vi "Modules Selector.vi"(6 "Scan All":bool, 10 "DQMH Modules":T1[](array[typedef]), 11 "Project In":refnum<class "Project.lvclass">) -> (3 "Project Out":refnum<class "Project.lvclass">, 4 "Scan?":bool)   [LabVIEW 2019, in "Panther Dashboard.lvlib" / "Project.lvclass"]
uses:
  Project.lvclass
  Panther Dashboard/Module to scan--cluster.ctl
  <vilib>/Delacor/Delacor QMH/Libraries/Scripting API/Module Information--cluster.ctl
  Panther Dashboard/Module type--enum.ctl
  Library/Library.lvclass
  Library/Library.lvclass/Library.ctl
  Project.lvclass/Project.ctl
  Library/Write Library Ref.vi
  Library/Write Type.vi
  Library/Write Library Description.vi
  Library/Write Dependency.vi
  Write Libraries.vi
  Panther Dashboard/Panther Dashboard.lvlib
  <vilib>/Delacor/Delacor QMH/Libraries/Scripting API/DQMH_Scripting API.lvlib
panel:
  in  "DQMH Modules found in Project":T2[](array[typedef])
  in  "Scan Selection":bool
  in  "Select/Unselect All":bool
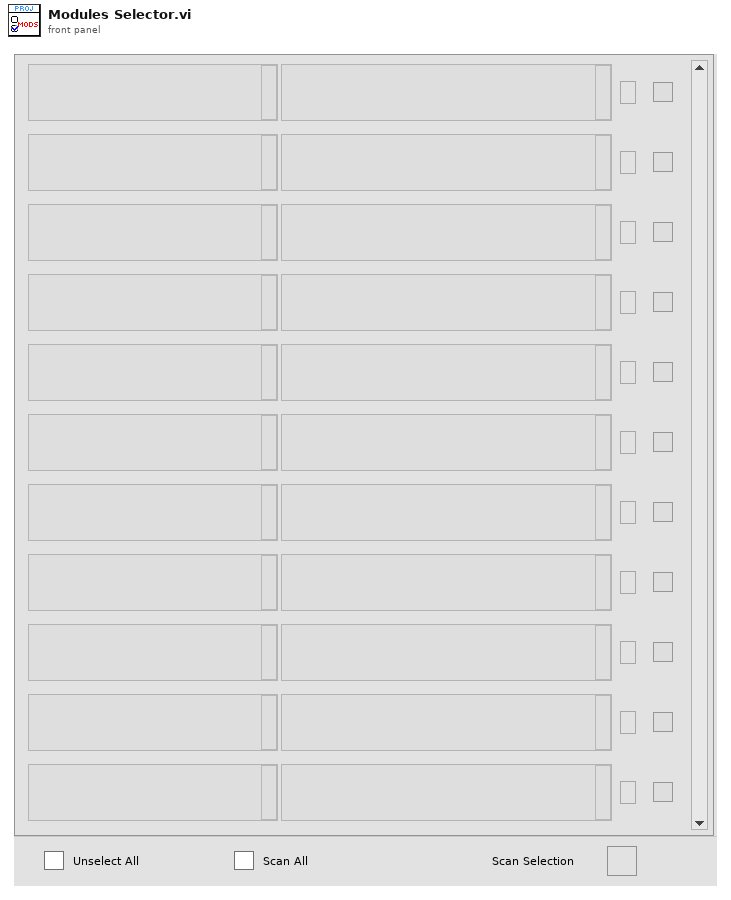
[diagram p1: front panel]
types:
  T1 = typedef "DQMH_Scripting API.lvlib/Module Information--cluster.ctl" = cluster{"Library":refnum<vi>, "Qualified Name":string, "Path":path, "Cloneable":bool, "Under Dependencies":bool}
  T2 = typedef "Panther Dashboard.lvlib/Module to scan--cluster.ctl" = cluster{"Module Name":string, "Description":string, "Scan?":bool, "Dependency":bool}
  T3 = typedef "Panther Dashboard.lvlib/Module type--enum.ctl" = enum16{"Singleton", "Cloneable"}
  T4 = enum32{"Invalid", "Standard", "Closed", "Hidden", "Minimized", "Maximized"}
  T5 = enum8{"Enabled", "Disabled", "Disabled and Grayed Out"}
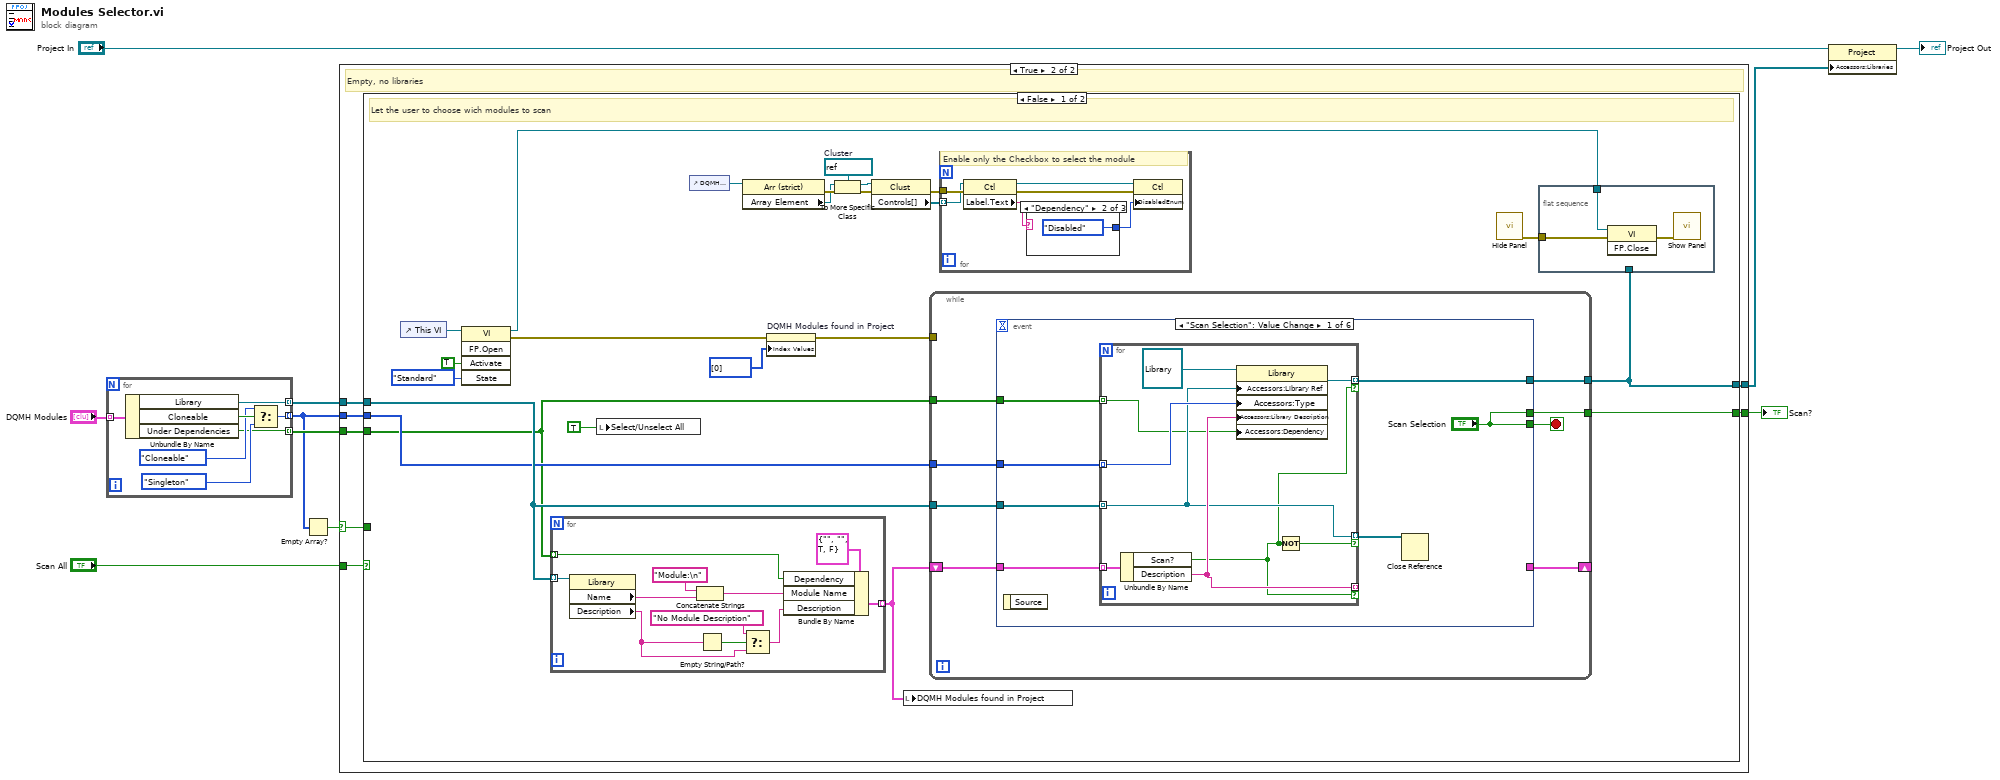
[diagram p0: block diagram]
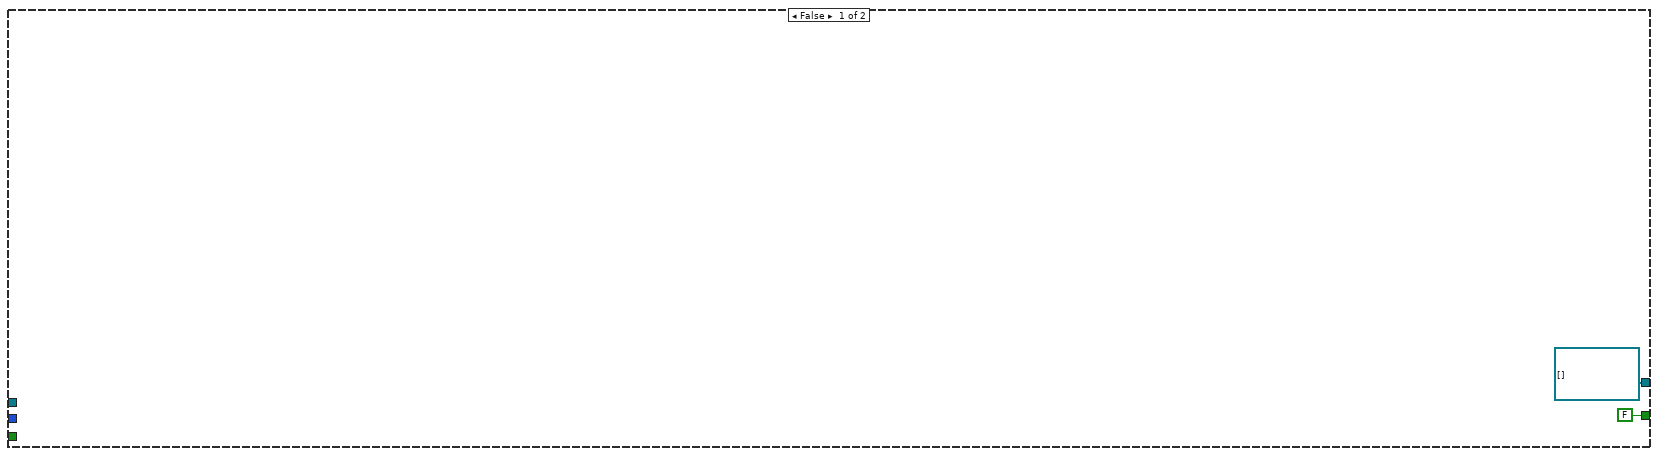
[diagram p2: hidden frame]
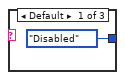
[diagram p3: hidden frame]
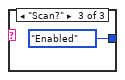
[diagram p4: hidden frame]
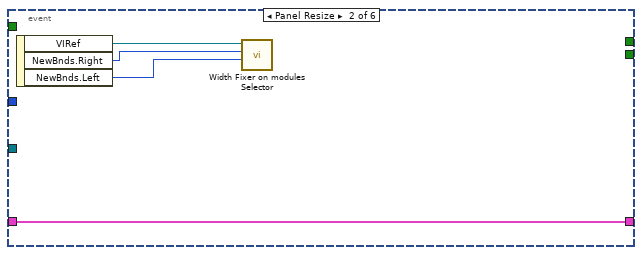
[diagram p5: hidden frame]
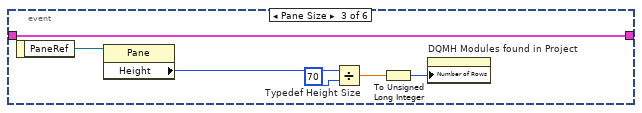
[diagram p6: hidden frame]
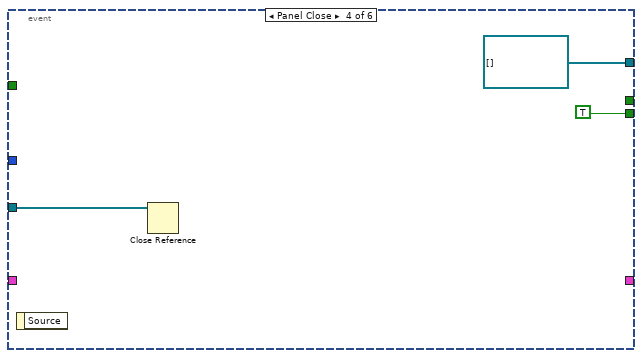
[diagram p7: hidden frame]
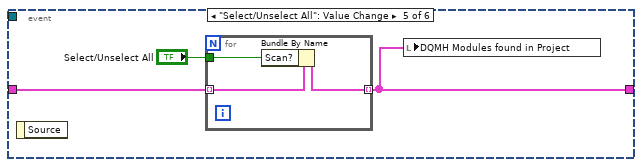
[diagram p8: hidden frame]
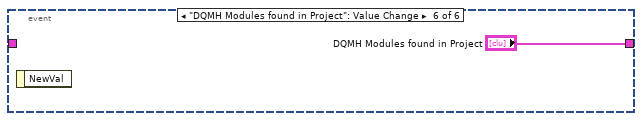
[diagram p9: hidden frame]
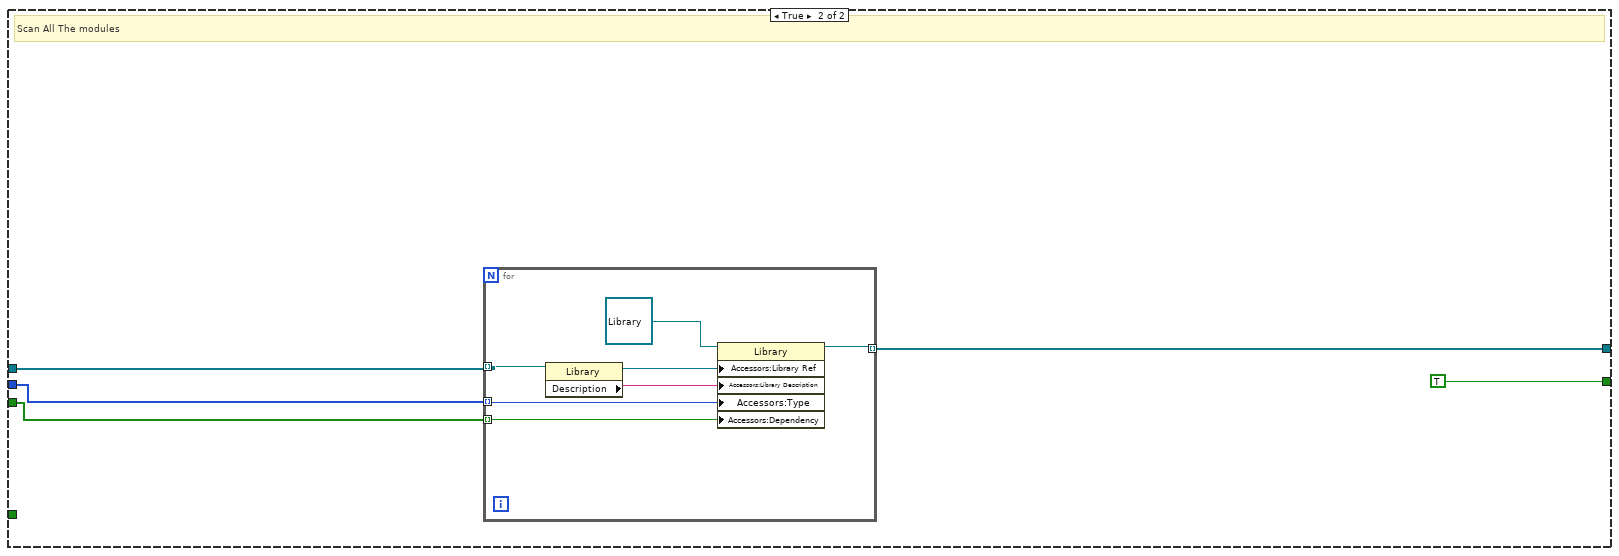
[diagram p10: hidden frame]
diagram:
  n1 = for {
    tunnel: "DQMH Modules" -> [w17] mode=indexing
    tunnel: [w16] -> w7 mode=indexing
    tunnel: [w12] -> w3 mode=indexing
    tunnel: [w11] -> w6 mode=indexing
    n2 = Unbundle By Name(w17) -> ("Library"=w16:refnum<vi>, "Cloneable"=w14:bool, "Under Dependencies"=w11:bool)
    n3 = Select(t=Module_type--enum."Cloneable", s=w14, f=Module_type--enum."Singleton" ("Module type")) -> (s? t:f=w12:T3)
  }
  n4 = Empty Array?(array=w3) -> (empty?=w4:bool)
  n5 = case shown="True" w4 {
    selector: w4 -> [_ w20]
    tunnel: [FALSE ("Scan Selection") w26] -> w10
    tunnel: "Scan All" -> [_ w25]
    tunnel: [refnum<class "Library.lvclass">[] [] w24] -> w8
    tunnel: w7 -> [_ w23]
    tunnel: w3 -> [_ w22]
    tunnel: w6 -> [_ w21]
    frame False {
    }
    frame True {
      # "Empty, no libraries"
      n6 = case shown="False" w25 {
        tunnel: w23 -> [w43 w120]
        tunnel: w22 -> [w42 w119]
        tunnel: w21 -> [w41 w118]
        tunnel: [w40 TRUE ("Scan Selection")] -> w26
        tunnel: [w27 w117] -> w24
        tunnel: w20 -> [_ _]
        frame False {
          w28 = refnum<vi> refnum  # Cluster
          # "Let the user to choose wich modules to scan"
          n7 = control-ref of="This VI"() -> (w39:refnum<vi>)
          n8 = invoke class="VI" method="FP.Open"(reference=w39, "Activate"=TRUE ("Activate?"), "State"=T4."Standard") -> (reference out=w36:refnum<vi>, error out=w49:errorcluster)  [unwired: 2 in, 3 out]
          n9 = for {
            tunnel: w43 -> [w72] mode=indexing
            tunnel: [w71] -> w35 mode=indexing
            tunnel: w41 -> [w62] mode=indexing
            n10 = property class="Library"(reference=w72) -> ("Name"=w69:string, "Description"=w67:string)  [unwired: 1 in, 2 out]
            n11 = Concatenate Strings("Module:\n" ("string"), w69) -> (w64:string)
            n12 = Empty String/Path?(string/path=w67) -> (empty?=w68:bool)
            n13 = Select(t="No Module Description", s=w68, f=w67) -> (s? t:f=w66:string)
            n14 = Bundle By Name(cluster=T2 {"Module Name"="", "Description"="", "Scan?"=TRUE, "Dependency"=FALSE} ("Module"), "Dependency"=w62, "Module Name"=w64, "Description"=w66) -> (w71:T2)
          }
          n15 = local write "Select/Unselect All"(TRUE ("Select /Unselect All Modules")) -> ()
          n16 = control-ref of="DQMH Modules found in Project"() -> (w29:refnum<vi>)
          n17 = property class="Arr (strict)"(reference=w29) -> (error out=w45:errorcluster, "Array Element"=w30:refnum<vi>)  [unwired: 1 in, 1 out]
          n18 = property on="DQMH Modules found in Project" class="Arr (strict)"(error in=w49, "Index Values"=u32[] [0]) -> (error out=w48:errorcluster)  [unwired: 1 in, 1 out]
          n19 = To More Specific Class(target class=w28, reference=w30, error in=w45) -> (specific class reference=w31:refnum<vi>, error out=w46:errorcluster)
          n20 = property class="Clust"(reference=w31, error in=w46) -> (error out=w47:errorcluster, "Controls[]"=w32:refnum<vi>[])  [unwired: 1 out]
          n21 = local write "DQMH Modules found in Project"(w35) -> ()
          n22 = while {
            shift-right: [w79] -> _
            shift-left: w35 -> [w80]
            tunnel: w43 -> [w78]
            tunnel: w42 -> [w77]
            tunnel: w48 -> [_]
            tunnel: w41 -> [w76]
            tunnel: [w74] -> w40
            tunnel: [w73] -> w27
            stop <- w75 stop-if-true
            n23 = event shown="[0] \"Scan Selection\": Value Change" {
              selector: _ -> [_ _ _ _ _ _]
              dyn-events: _ -> [_ _ _ _ _ _]
              timeout: _ -> [_ _ _ _ _ _]
              tunnel: w80 -> [w87 w100 w102 _ w112 _]
              tunnel: ["Scan Selection" _ _ TRUE ("All") _ _] -> w75
              tunnel: [_ w100 w102 _ w111 "DQMH Modules found in Project"] -> w79
              tunnel: w78 -> [w85 _ _ w108 _ _]
              tunnel: w77 -> [w86 _ _ _ _ _]
              tunnel: w76 -> [w83 _ _ _ _ _]
              tunnel: ["Scan Selection" _ _ _ _ _] -> w74
              tunnel: [w81 _ _ refnum<class "Library.lvclass">[] [] _ _] -> w73
              event "Scan Selection": Value Change {
                n24 = event-data() -> ()  [unwired: 1 in, 1 out]
                n25 = for {
                  tunnel: w87 -> [w96] mode=indexing
                  tunnel: [w92] -> _ mode=indexing if=w88
                  tunnel: w86 -> [w91] mode=indexing
                  tunnel: w85 -> [w90] mode=indexing
                  tunnel: [w90] -> w84 mode=indexing if=w95
                  tunnel: w83 -> [w89] mode=indexing
                  tunnel: [w93] -> w81 mode=indexing if=w88
                  n26 = Unbundle By Name(w96) -> ("Scan?"=w88:bool, "Description"=w92:string)
                  n27 = property class="Library"(reference=refnum<class "Library.lvclass"> refnum ("Library.lvclass"), "Accessors:Library Ref"=w90, "Accessors:Type"=w91, "Accessors:Library Description"=w92, "Accessors:Dependency"=w89) -> (reference out=w93:refnum<class "Library.lvclass">)  [unwired: 1 in, 1 out]
                  n28 = Not(x=w88) -> (.not. x?=w95:bool)
                }
                n29 = Close Reference(reference=w84) -> ()  [unwired: 1 in, 1 out]
              }
              event Panel Resize {
                n30 = event-data() -> ("VIRef"=w99:refnum<vi>, "NewBnds.Right"=w97:i16, "NewBnds.Left"=w98:i16)  [unwired: 1 in]
                n31 = call "Width Fixer on modules Selector.vi"("Left"=w98, "Right"=w97, "VI in"=w99) -> ()  [unwired: 9 in]
              }
              event Pane Size {
                w104 = u32 70  # Typedef Height Size
                n32 = event-data() -> ("PaneRef"=w106:refnum<vi>)  [unwired: 1 in]
                n33 = property class="Pane"(reference=w106) -> ("Height"=w105:u32)  [unwired: 1 in, 2 out]
                n34 = Divide(x=w105, y=w104) -> (x/y=w103:dbl)
                n35 = To Unsigned Long Integer(number=w103) -> (unsigned 32bit integer=w101:u32)
                n36 = property on="DQMH Modules found in Project" class="Arr (strict)"("Number of Rows"=w101) -> ()  [unwired: 2 in, 2 out]
              }
              event Panel Close {
                n37 = event-data() -> ()  [unwired: 1 in, 1 out]
                n38 = Close Reference(reference=w108) -> ()  [unwired: 1 in, 1 out]
              }
              event "Select/Unselect All": Value Change {
                n39 = event-data() -> ()  [unwired: 1 in, 1 out]
                n40 = for {
                  tunnel: w112 -> [w115] mode=indexing
                  tunnel: [w114] -> w111 mode=indexing
                  tunnel: "Select/Unselect All" -> [w113]
                  n41 = Bundle By Name(cluster=w115, "Scan?"=w113) -> (w114:T2)
                }
                n42 = local write "DQMH Modules found in Project"(w111) -> ()
              }
              event "DQMH Modules found in Project": Value Change {
                n43 = event-data() -> ()  [unwired: 1 in, 1 out]
              }
            }
          }
          n44 = for {
            tunnel: w32 -> [w56] mode=indexing
            tunnel: w47 -> [w58]
            # "Enable only the Checkbox to select the module"
            n45 = property class="Ctl"(reference=w56, error in=w58) -> (reference out=w54:refnum<vi>, error out=w57:errorcluster, "Label.Text"=w55:string)
            n46 = case shown="\"Dependency\"" w55 {
              tunnel: [T5."Disabled" ("Disabled") T5."Disabled" ("Disabled") T5."Enabled" ("Disabled")] -> w53
              frame Default {
              }
              frame "Dependency" {
              }
              frame "Scan?" {
              }
            }
            n47 = property class="Ctl"(reference=w54, error in=w57, "DisabledEnum"=w53) -> ()  [unwired: 2 out]
          }
          n48 = call "Hide Panel.vi"() -> ("error out"=w44:errorcluster)  [unwired: 11 in]
          n49 = flat-sequence {
            tunnel: w36 -> [w50]
            tunnel: w27 -> [_]
            tunnel: w44 -> [w51]
            frame #0 {
              n50 = invoke class="VI" method="FP.Close"(reference=w50, error in=w51) -> (error out=w52:errorcluster)  [unwired: 1 in, 2 out]
              n51 = call "Show Panel.vi"("error in (no error)"=w52) -> ()  [unwired: 10 in, 1 out]
            }
          }
        }
        frame True {
          # "Scan All The modules"
          n52 = for {
            tunnel: w120 -> [w127] mode=indexing
            tunnel: w119 -> [w126] mode=indexing
            tunnel: w118 -> [w125] mode=indexing
            tunnel: [w124] -> w117 mode=indexing
            n53 = property class="Library"(reference=w127) -> (reference out=w122:refnum<vi>, "Description"=w123:string)  [unwired: 1 in, 1 out]
            n54 = property class="Library"(reference=refnum<class "Library.lvclass"> refnum ("Library.lvclass"), "Accessors:Library Ref"=w122, "Accessors:Library Description"=w123, "Accessors:Type"=w126, "Accessors:Dependency"=w125) -> (reference out=w124:refnum<class "Library.lvclass">)  [unwired: 1 in, 1 out]
          }
        }
      }
    }
  }
  "Scan?" <- w10
  n55 = property class="Project"(reference="Project In", "Accessors:Libraries"=w8) -> (reference out=→"Project Out":refnum<class "Project.lvclass">)  [unwired: 1 in, 1 out]
